vi "Close Wrapper.vi"(8 "error in (no error)":errorcluster, 11 "Session":u64) -> (0 "error out":errorcluster)   [LabVIEW 2021, in "Zenoh.lvclass"]
uses:
  Zenoh.lvclass
  Zenoh.lvclass/Zenoh.ctl
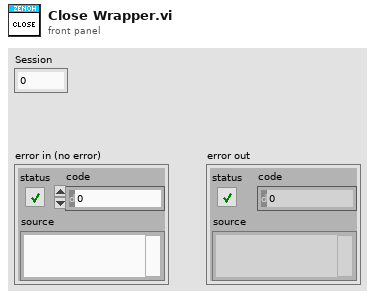
[diagram p1: front panel]
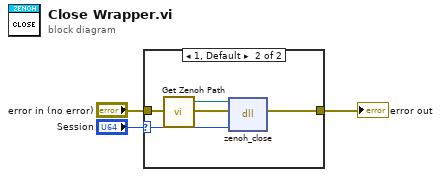
[diagram p0: block diagram]
diagram:
  n1 = case shown="1, Default" "Session" {
    selector: "Session" -> [_ w5]
    tunnel: "error in (no error)" -> [w4 w7]
    tunnel: [w4 w6] -> w2
    frame 0 {
    }
    frame 1, Default {
      n2 = call "Get Zenoh Path.vi"() -> ("Library Path"=w8:path)  [unwired: 4 in]
      n3 = dll-call lib="C:/Program Files/CIF_Foundation/Libraries/zenoh_lv_wrapper.dll" fn="zenoh_close"(path in=w8, error in=w7, "session_ptr"=w5) -> (error out=w6:errorcluster)  [unwired: 3 in, 1 out]
    }
  }
  "error out" <- w2
